vi "Module - Network Stream.vi"(8 "error in (no error)":errorcluster) -> (0 "error out":errorcluster)   [LabVIEW 2020]
uses:
  Control/State - Network Stream.ctl
  Control/State - eFGV.ctl
  Control/Section Config RT.ctl
  <vilib>/dex/Flush And Wait Empty Condition.ctl
  <vilib>/Utility/error.llb/DialogType.ctl
  <resource>/objmgr/ni.dex.rc
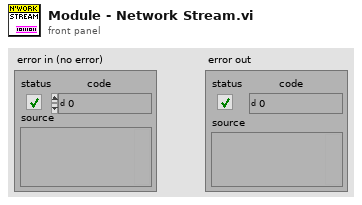
[diagram p1: front panel]
types:
  T1 = cluster{"TOut":i32, "Stream connected?":bool, "User exit":bool, "Module Name":string, "writer endpoint":refnum<k21>, "timeout in ms (-1)":i32, "writer buffer size":i32, "writer name":string, "Rotaton Angle":sgl, "AI Calibrated Data":sgl[], "Event Ref":refnum<event-registration>}
  T2 = typedef "State - Network Stream.ctl" = enum16{"Init module", "Register for event", "Read Config File", "Idle", "Create writer endpoint", "Send data to stream", "Check stream conn", "Destroy endpoint", "Unregister user event", "Close module"}
  T3 = typedef "Section Config RT.ctl" = enum16{"Mod1/AI0", "Mod1/AI1", "Mod1/AI2", "Mod1/AI3", "Network Stream", "Acquisition Setting"}
  T4 = cluster{"Data Name":string, "Data Value":variant}
  T5 = typedef "State - eFGV.ctl" = enum16{"Init", "Read", "Write", "Exit"}
  T6 = typedef "Flush And Wait Empty Condition.ctl" = u8
  T7 = typedef "DialogType.ctl" = u16
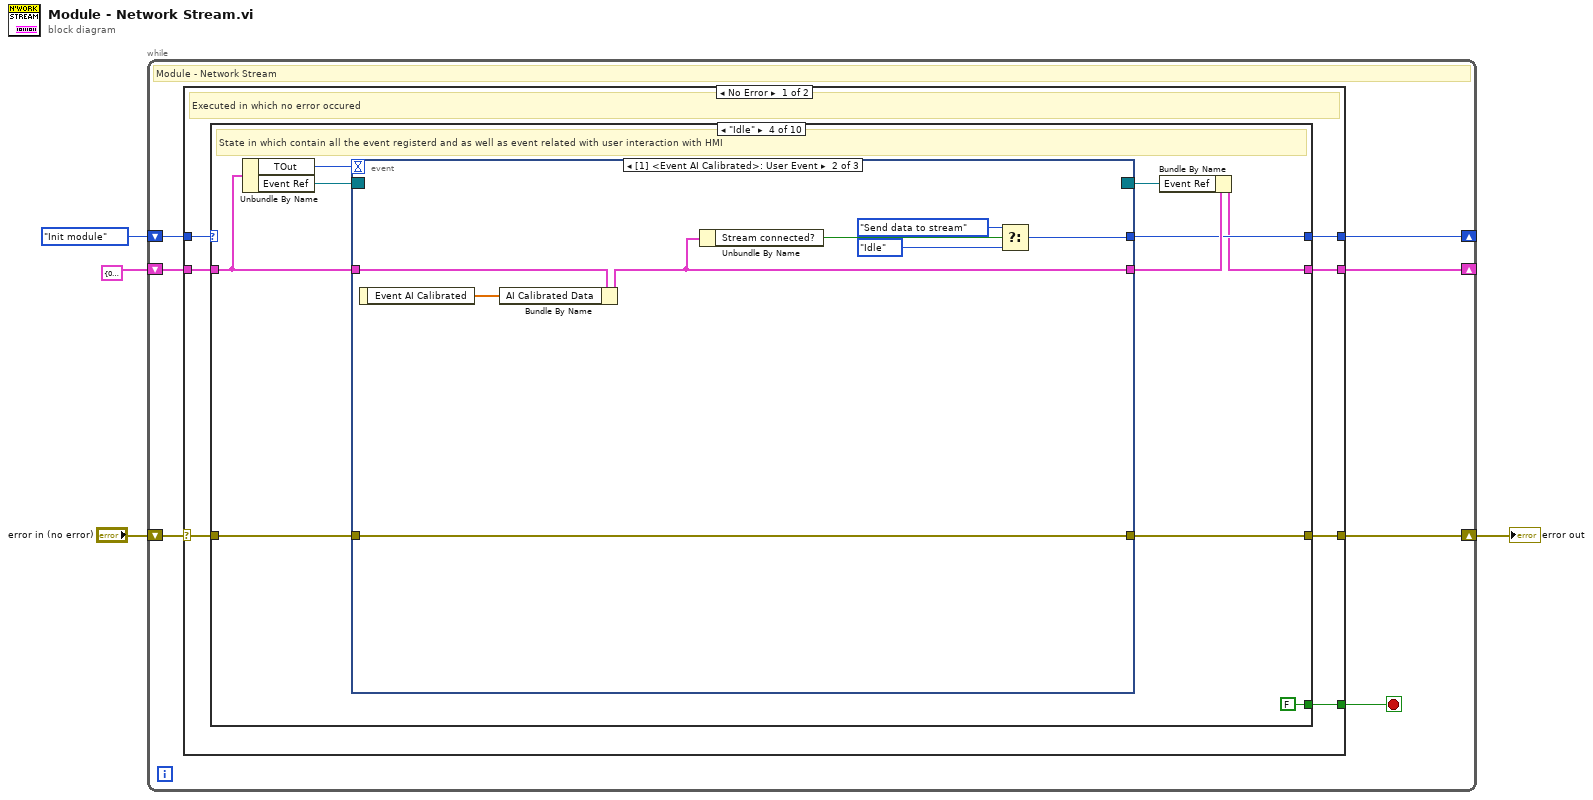
[diagram p0: block diagram]
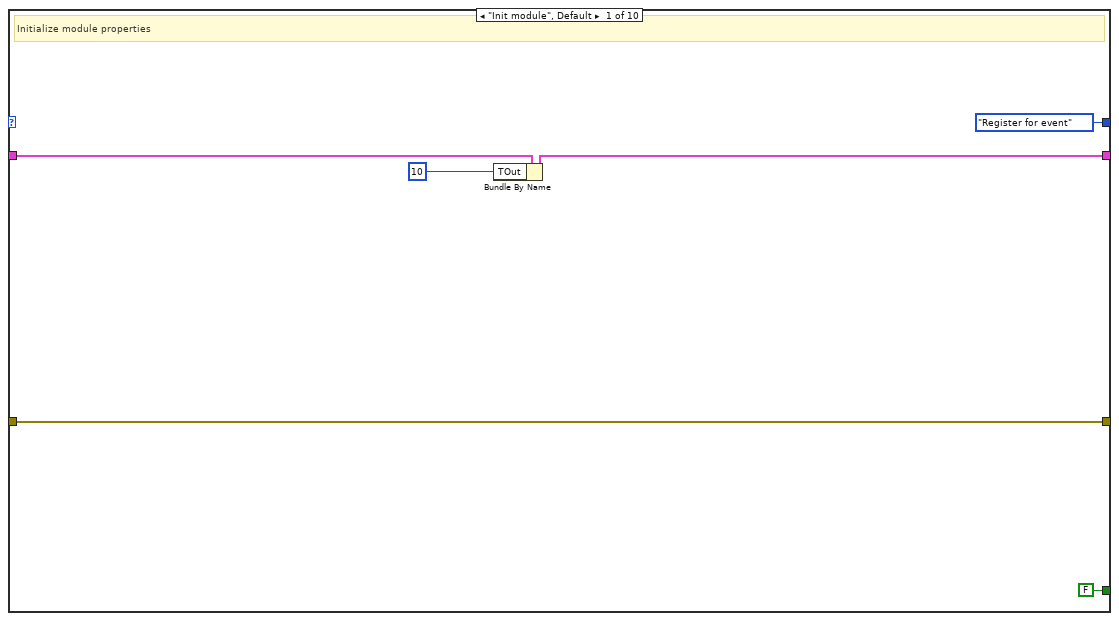
[diagram p2: hidden frame]
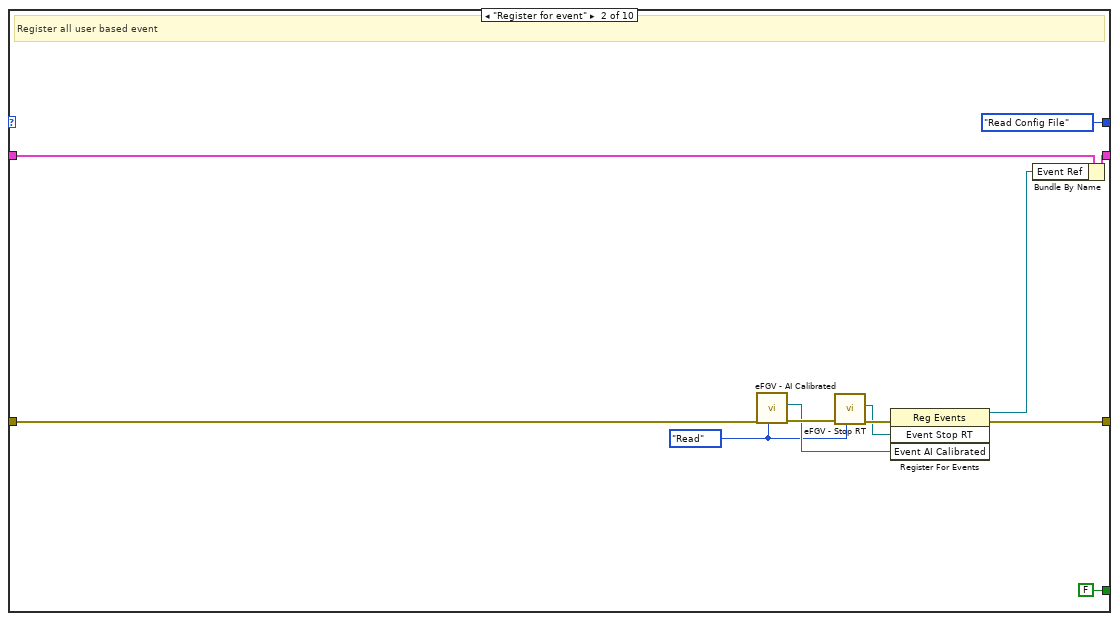
[diagram p3: hidden frame]
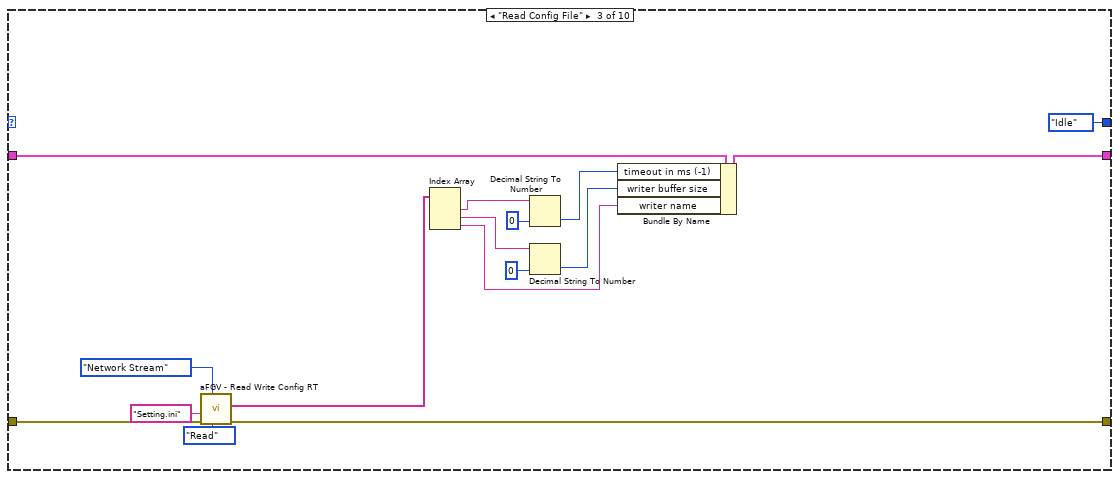
[diagram p4: hidden frame]
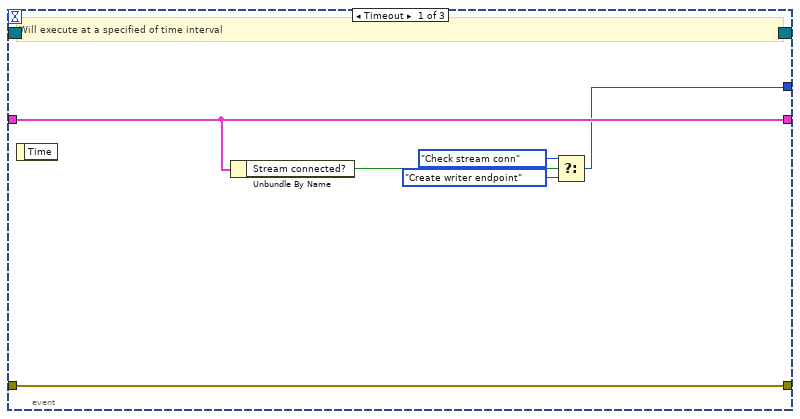
[diagram p5: hidden frame]
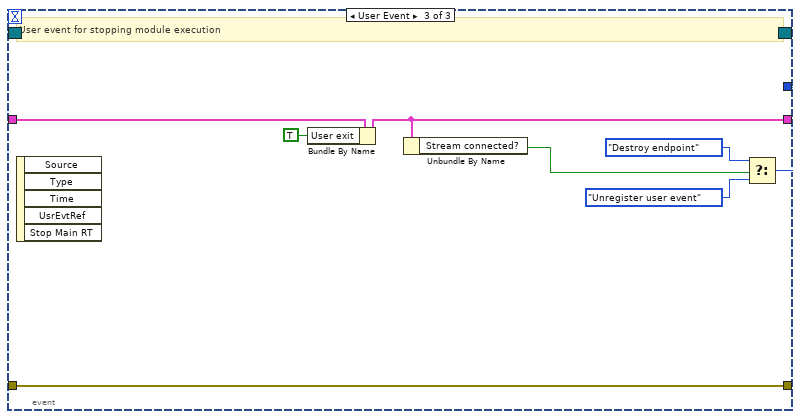
[diagram p6: hidden frame]
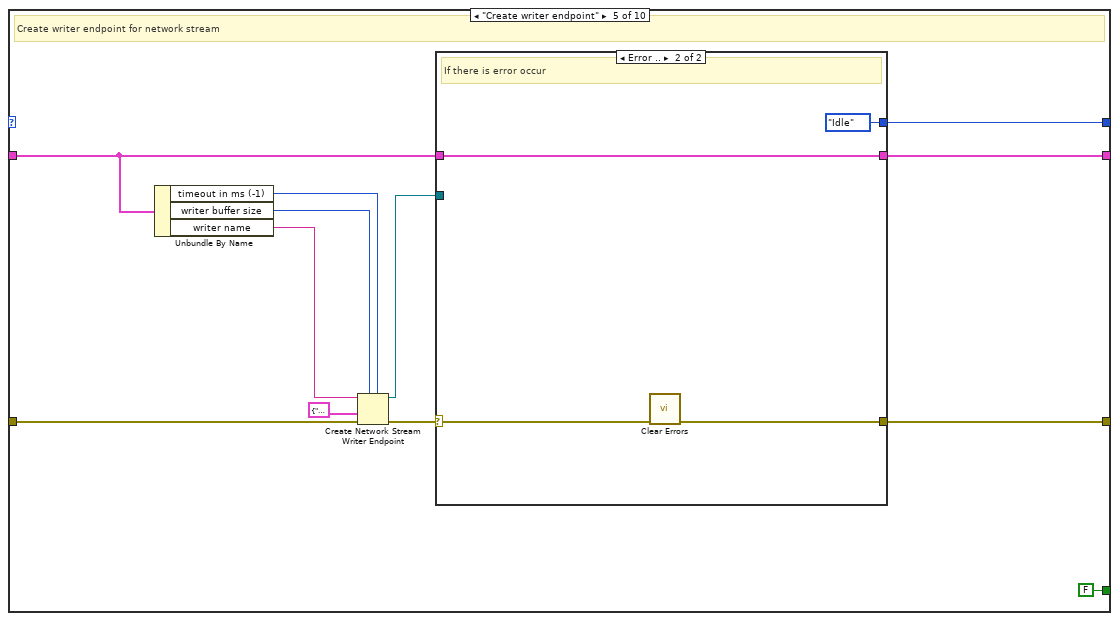
[diagram p7: hidden frame]
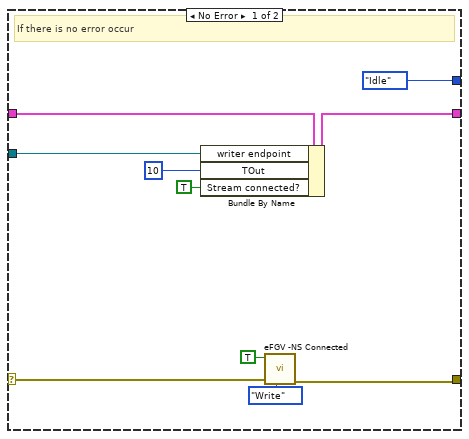
[diagram p8: hidden frame]
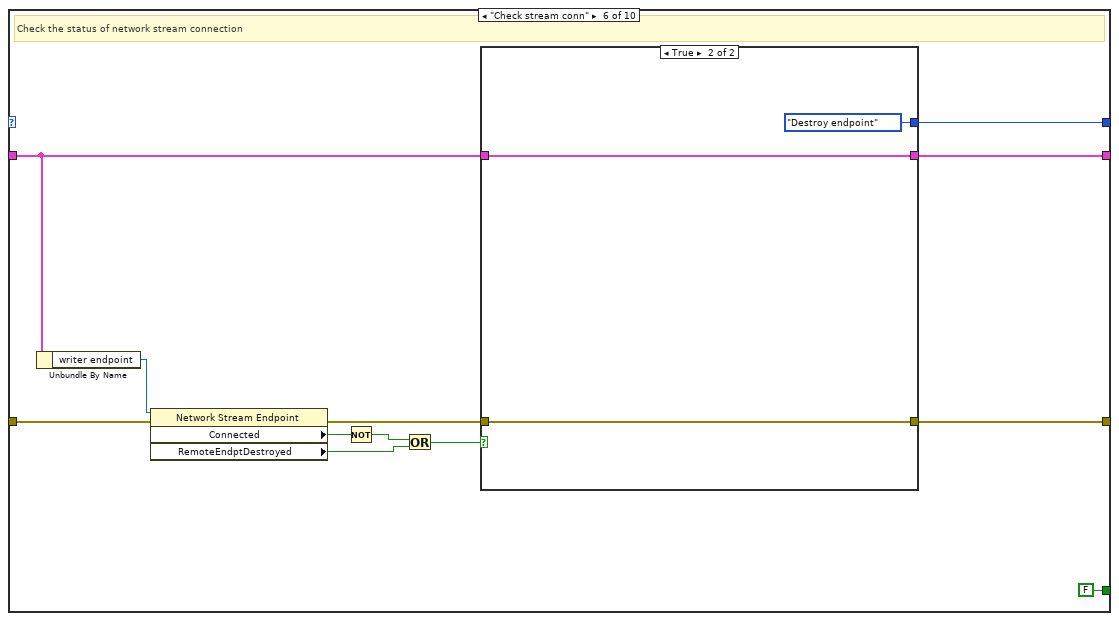
[diagram p9: hidden frame]
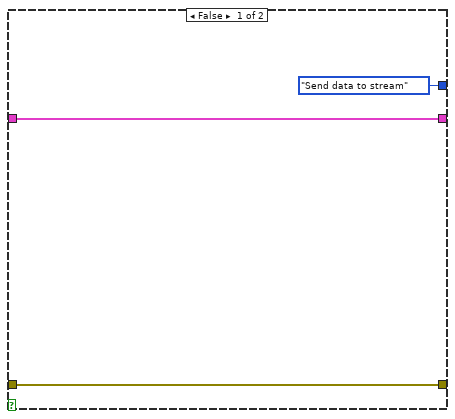
[diagram p10: hidden frame]
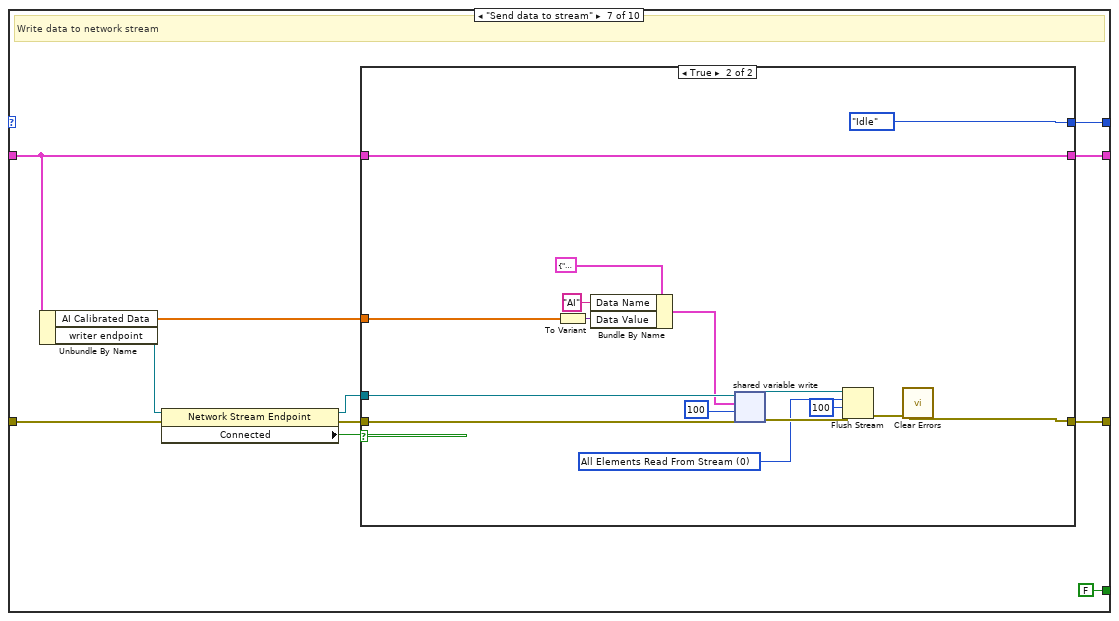
[diagram p11: hidden frame]
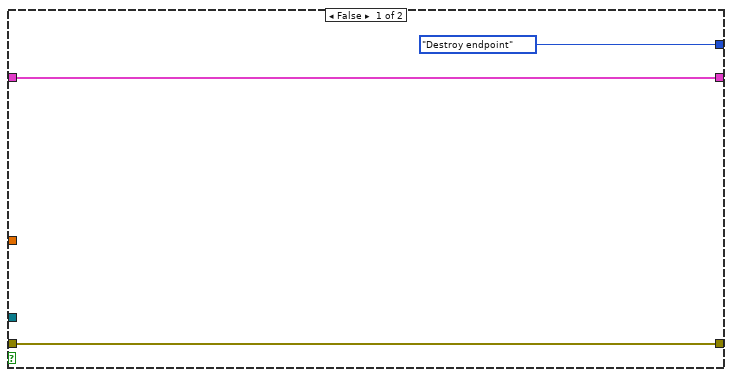
[diagram p12: hidden frame]
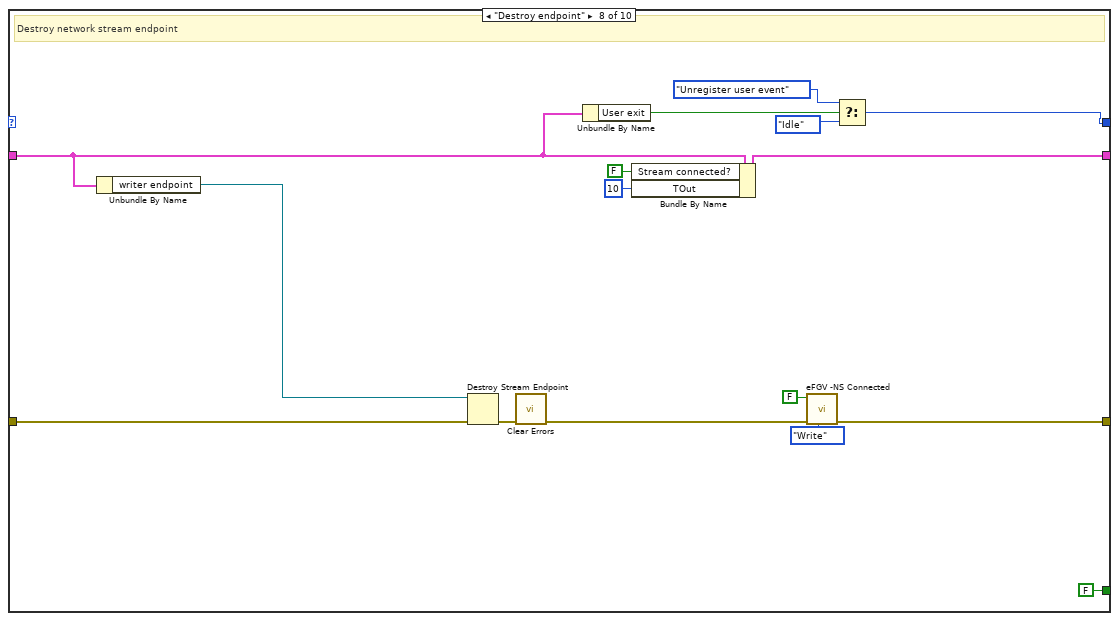
[diagram p13: hidden frame]
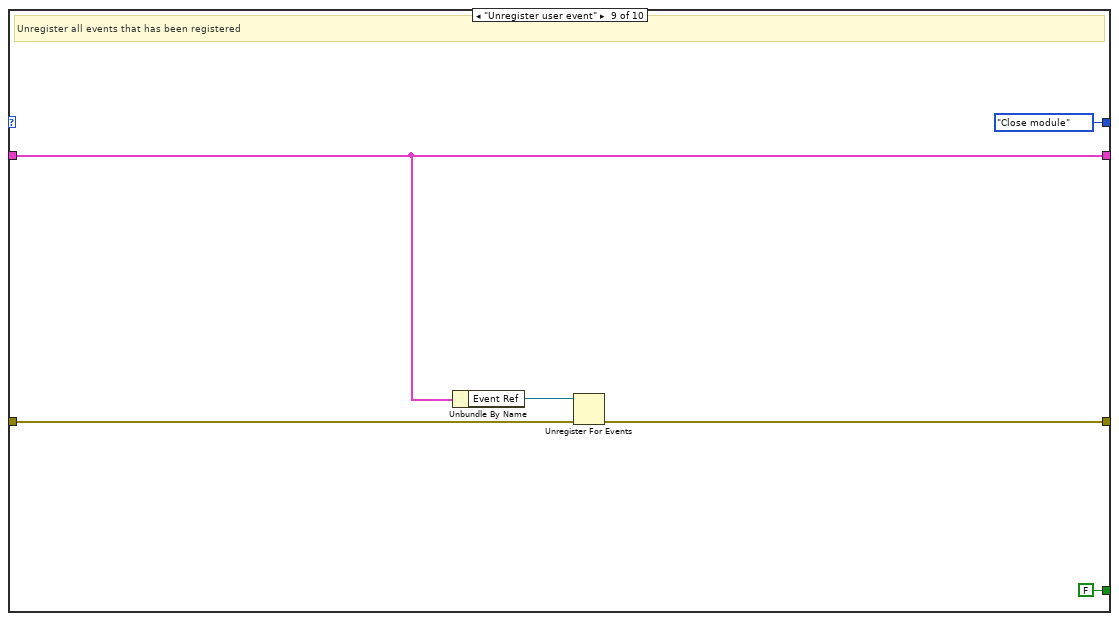
[diagram p14: hidden frame]
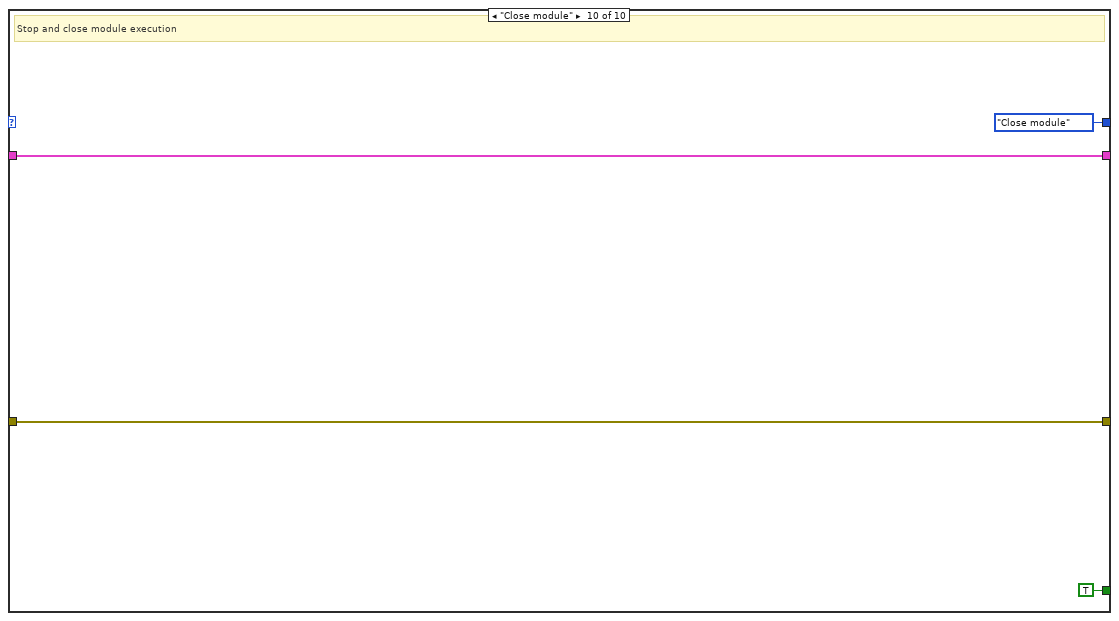
[diagram p15: hidden frame]
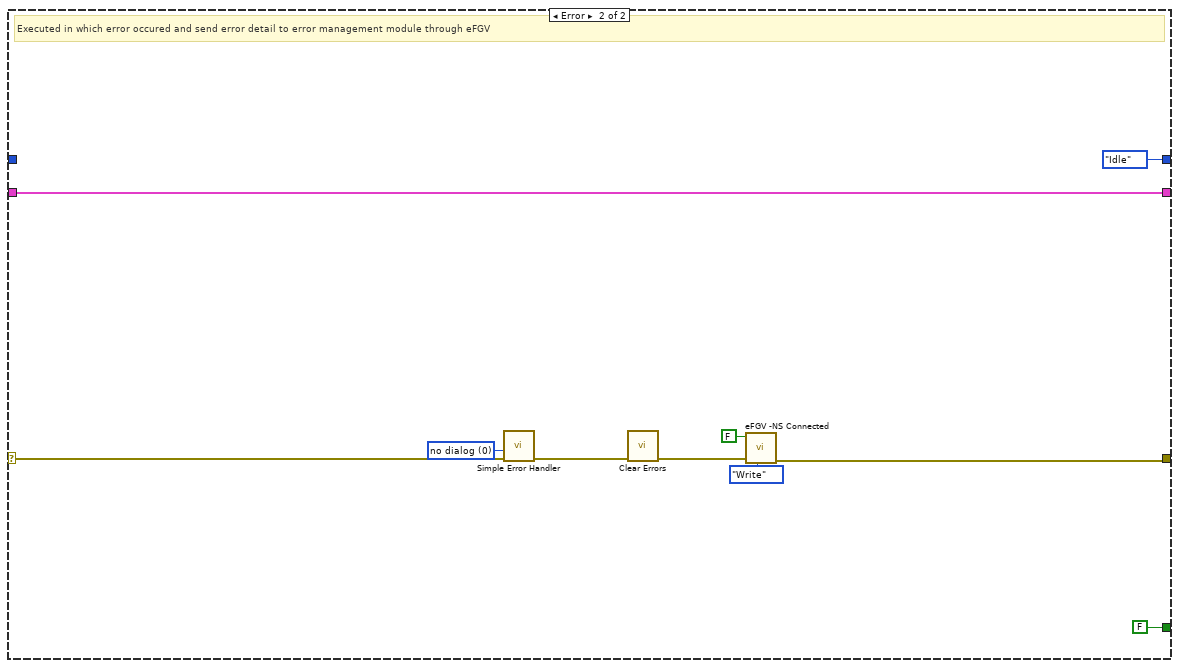
[diagram p16: hidden frame]
diagram:
  n1 = while {
    shift-right: [w7] -> w3
    shift-left: "error in (no error)" -> [w11]
    shift-right: [w5] -> _
    shift-left: State_-_Network_Stream."Init module" -> [w9]
    shift-right: [w6] -> _
    shift-left: T1 {"TOut"=0, "Stream connected?"=FALSE, "User exit"=FALSE, "Module Name"="", "writer endpoint"="", "timeout in ms (-1)"=3000, "writer buffer size"=20, "writer name"="EngineStream", "Rotaton Angle"=0.0, "AI Calibrated Data"=[0.0, 0.0, 0.0, 0.0], "Event Ref"=refnum} -> [w8]
    stop <- w10 stop-if-true
    # "Module - Network Stream"
    n2 = case shown="No Error" w11 {
      selector: w11 -> [w18 w193]
      tunnel: [w17 FALSE] -> w10
      tunnel: w9 -> [w16 _]
      tunnel: w8 -> [w15 w191]
      tunnel: [w14 w185] -> w7
      tunnel: [w13 w191] -> w6
      tunnel: [w12 State_-_Network_Stream."Idle"] -> w5
      frame No Error {
        # "Executed in which no error occured"
        n3 = case shown="\"Idle\"" w16 {
          tunnel: w18 -> [w19 w30 w42 w62 w95 w118 w135 w168 w177 w184]
          tunnel: [FALSE FALSE _ FALSE FALSE FALSE FALSE FALSE FALSE TRUE] -> w17
          tunnel: w15 -> [w23 w34 w52 w59 w88 w120 w137 w170 w176 w183]
          tunnel: [w19 w35 w41 w61 w94 w121 w138 w159 w180 w184] -> w14
          tunnel: [w21 w26 w51 w54 w93 w115 w134 w166 w176 w183] -> w13
          tunnel: [State_-_Network_Stream."Register for event" State_-_Network_Stream."Read Config File" State_-_Network_Stream."Idle" w56 w90 w119 w136 w171 State_-_Network_Stream."Close module" State_-_Network_Stream."Close module"] -> w12
          frame "Init module", Default {
            # "Initialize module properties"
            n4 = Bundle By Name(cluster=w23, "TOut"=10) -> (w21:T1)
          }
          frame "Register for event" {
            w27 = State_-_eFGV."Read" ("State")
            # "Register all user based event"
            n5 = call "eFGV - AI Calibrated.vi"("State"=w27, "error in (no error)"=w30) -> ("error out"=w29:errorcluster, "Event AI Calibrated"=w28:refnum<user-event>)  [unwired: 8 in]
            n6 = call "eFGV - Stop RT.vi"("State"=w27, "Error In"=w29) -> ("Error Out"=w32:errorcluster, "Event Stop RT"=w31:refnum<user-event>)  [unwired: 7 in, 1 out]
            n7 = register-events(error in=w32, w31, w28) -> (reference out=w25:refnum<event-registration>, error out=w35:errorcluster)  [unwired: 1 in]
            n8 = Bundle By Name(cluster=w34, "Event Ref"=w25) -> (w26:T1)
          }
          frame "Read Config File" {
            n9 = call "aFGV - Read Write Config RT.vi"("State"=enum16{"Read", "Write", "Delete"}."Read", "Section"=Section_Config_RT."Network Stream", "Error In"=w42, "File name"="Setting.ini") -> ("Error Out"=w41:errorcluster, "Data out"=w40:string[])  [unwired: 5 in, 1 out]
            n10 = Index Array(array=w40) -> (element #1=w50:string, element #2=w49:string, element #3=w44:string)  [unwired: 3 in]
            n11 = Decimal String To Number(string=w50, default (0L)=0 ("timeout in ms (-1)")) -> (number=w46:i32)  [unwired: 1 in, 1 out]
            n12 = Decimal String To Number(string=w49, default (0L)=0 ("writer buffer size")) -> (number=w45:i32)  [unwired: 1 in, 1 out]
            n13 = Bundle By Name(cluster=w52, "timeout in ms (-1)"=w46, "writer buffer size"=w45, "writer name"=w44) -> (w51:T1)
          }
          frame "Idle" {
            # "State in which contain all the event registerd and as well as event related with user interaction with HMI"
            n14 = Unbundle By Name(w59) -> ("TOut"=w60:i32, "Event Ref"=w55:refnum<event-registration>)
            n15 = event shown="[1] <Event AI Calibrated>: User Event" {
              selector: w55 -> [_ _ _]
              dyn-events: [_ _ _] -> w53
              timeout: w60 -> [_ _ _]
              tunnel: w62 -> [w68 w69 w84]
              tunnel: [w68 w69 w84] -> w61
              tunnel: w59 -> [w67 w76 w83]
              tunnel: [w67 w71 w81] -> w58
              tunnel: [w63 w72 w77] -> w56
              event Timeout {
                # "Will execute at a specified of time interval"
                n16 = event-data() -> ()  [unwired: 1 in, 1 out]
                n17 = Unbundle By Name(w67) -> ("Stream connected?"=w66:bool)
                n18 = Select(t=State_-_Network_Stream."Check stream conn", s=w66, f=State_-_Network_Stream."Create writer endpoint") -> (s? t:f=w63:T2)
              }
              event User Event {
                n19 = event-data() -> ("Event AI Calibrated"=w70:sgl[])  [unwired: 1 in]
                n20 = Bundle By Name(cluster=w76, "AI Calibrated Data"=w70) -> (w71:T1)
                n21 = Unbundle By Name(w71) -> ("Stream connected?"=w75:bool)
                n22 = Select(t=State_-_Network_Stream."Send data to stream", s=w75, f=State_-_Network_Stream."Idle") -> (s? t:f=w72:T2)
              }
              event User Event {
                # "User event for stopping module execution"
                n23 = event-data() -> ()  [unwired: 1 in, 5 out]
                n24 = Bundle By Name(cluster=w83, "User exit"=TRUE) -> (w81:T1)
                n25 = Unbundle By Name(w81) -> ("Stream connected?"=w80:bool)
                n26 = Select(t=State_-_Network_Stream."Destroy endpoint", s=w80, f=State_-_Network_Stream."Unregister user event") -> (s? t:f=w77:T2)
              }
            }
            n27 = Bundle By Name(cluster=w58, "Event Ref"=w53) -> (w54:T1)
          }
          frame "Create writer endpoint" {
            # "Create writer endpoint for network stream"
            n28 = Unbundle By Name(w88) -> ("timeout in ms (-1)"=w87:i32, "writer buffer size"=w86:i32, "writer name"=w85:string)
            n29 = Create Network Stream Writer Endpoint(5:w87, 7:w86, 8:w95, 9:T4 {"Data Name"="", "Data Value"=variant}, 11:w85) -> (0:w91:errorcluster, 3:w92:refnum<k21>)  [unwired: 2 in]
            n30 = case shown="Error .." w91 {
              selector: w91 -> [w98 w108]
              tunnel: w88 -> [w106 w110]
              tunnel: [w97 w109] -> w94
              tunnel: [w105 w110] -> w93
              tunnel: w92 -> [w101 _]
              tunnel: [State_-_Network_Stream."Idle" State_-_Network_Stream."Idle"] -> w90
              frame No Error {
                # "If there is no error occur"
                n31 = Bundle By Name(cluster=w106, "writer endpoint"=w101, "TOut"=10, "Stream connected?"=TRUE) -> (w105:T1)
                n32 = call "eFGV -NS Connected.vi"("States"=State_-_eFGV."Write" ("State"), "Error In"=w98, "NS Connected"=TRUE) -> ("Error Out"=w97:errorcluster)  [unwired: 7 in, 1 out]
              }
              frame Error {
                # "If there is error occur"
                n33 = call <vilib>:"Clear Errors.vi"("error in (no error)"=w108) -> ("error out"=w109:errorcluster)  [unwired: 5 in, 1 out]
              }
            }
          }
          frame "Check stream conn" {
            # "Check the status of network stream connection"
            n34 = Unbundle By Name(w120) -> ("writer endpoint"=w117:refnum<k21>)
            n35 = property class="Network Stream Endpoint"(reference=w117, error in=w118) -> (error out=w116:errorcluster, "Connected"=w114:bool, "RemoteEndptDestroyed"=w113:bool)  [unwired: 1 out]
            n36 = Not(x=w114) -> (.not. x?=w111:bool)
            n37 = Or(x=w111, y=w113) -> (x .or. y?=w112:bool)
            n38 = case shown="True" w112 {
              tunnel: w116 -> [w125 w128]
              tunnel: [w125 w128] -> w121
              tunnel: w120 -> [w124 w127]
              tunnel: [State_-_Network_Stream."Send data to stream" State_-_Network_Stream."Destroy endpoint"] -> w119
              tunnel: [w124 w127] -> w115
              frame False {
              }
              frame True {
              }
            }
          }
          frame "Send data to stream" {
            # "Write data to network stream"
            n39 = Unbundle By Name(w137) -> ("AI Calibrated Data"=w129:sgl[], "writer endpoint"=w133:refnum<k21>)
            n40 = property class="Network Stream Endpoint"(reference=w133, error in=w135) -> (reference out=w130:refnum<k21>, error out=w132:errorcluster, "Connected"=w131:bool)
            n41 = case shown="True" w131 {
              tunnel: w132 -> [w142 w156]
              tunnel: [w142 w154] -> w138
              tunnel: w137 -> [w141 w155]
              tunnel: [State_-_Network_Stream."Destroy endpoint" State_-_Network_Stream."Idle"] -> w136
              tunnel: [w141 w155] -> w134
              tunnel: w130 -> [_ w157]
              tunnel: w129 -> [_ w144]
              frame False {
              }
              frame True {
                w146 = T6 0 items=["All Elements Read From Stream", "All Elements Available for Reading"] ("wait condition")
                n42 = To Variant(anything=w144) -> (Variant=w145:variant)
                n43 = Bundle By Name(cluster=T4 {"Data Name"="", "Data Value"=variant} ("data in"), "Data Name"="AI", "Data Value"=w145) -> (w152:T4)
                n44 = shared-variable-write(w157, w156, w152, 100 ("timeout ms (-1)")) -> (w147:refnum<k21>, w149:errorcluster)  [unwired: 1 out]
                n45 = Flush Stream(8:w149, 9:100 ("timeout in ms (-1)"), 10:w146, 11:w147) -> (0:w148:errorcluster)  [unwired: 2 out]
                n46 = call <vilib>:"Clear Errors.vi"("error in (no error)"=w148) -> ("error out"=w154:errorcluster)  [unwired: 5 in, 1 out]
              }
            }
          }
          frame "Destroy endpoint" {
            # "Destroy network stream endpoint"
            n47 = Unbundle By Name(w170) -> ("writer endpoint"=w167:refnum<k21>)
            n48 = Destroy Stream Endpoint(8:w168, 11:w167) -> (0:w169:errorcluster)
            n49 = call <vilib>:"Clear Errors.vi"("error in (no error)"=w169) -> ("error out"=w161:errorcluster)  [unwired: 5 in, 1 out]
            n50 = Unbundle By Name(w170) -> ("User exit"=w174:bool)
            n51 = Bundle By Name(cluster=w170, "Stream connected?"=FALSE, "TOut"=10) -> (w166:T1)
            n52 = call "eFGV -NS Connected.vi"("States"=State_-_eFGV."Write" ("State"), "Error In"=w161, "NS Connected"=FALSE) -> ("Error Out"=w159:errorcluster)  [unwired: 7 in, 1 out]
            n53 = Select(t=State_-_Network_Stream."Unregister user event", s=w174, f=State_-_Network_Stream."Idle") -> (s? t:f=w171:T2)
          }
          frame "Unregister user event" {
            # "Unregister all events that has been registered"
            n54 = Unbundle By Name(w176) -> ("Event Ref"=w175:refnum<event-registration>)
            n55 = Unregister For Events(event registration refnum=w175, error in=w177) -> (error out=w180:errorcluster)
          }
          frame "Close module" {
            # "Stop and close module execution"
          }
        }
      }
      frame Error {
        w189 = T7 0 items=["no dialog", "OK message", "continue or stop message", "OK message + warnings", "continue/stop + warnings"] ("type of dialog (OK msg:1)")
        # "Executed in which error occured and send error detail to error management module through eFGV"
        n56 = call <vilib>:"Simple Error Handler.vi"("type of dialog (OK msg:1)"=w189, "error in (no error)"=w193) -> ("error out"=w192:errorcluster)  [unwired: 3 in, 4 out]
        n57 = call <vilib>:"Clear Errors.vi"("error in (no error)"=w192) -> ("error out"=w186:errorcluster)  [unwired: 5 in, 1 out]
        n58 = call "eFGV -NS Connected.vi"("States"=State_-_eFGV."Write" ("State"), "Error In"=w186, "NS Connected"=FALSE) -> ("Error Out"=w185:errorcluster)  [unwired: 7 in, 1 out]
      }
    }
  }
  "error out" <- w3
